vi "ChiSquareCalculation.vi"(2 "Extinction ExtinctionUncertainity Size parameter and Number ofS sizes 2":T2={"Extinction"=[], "Extinction Uncertainty"=[], "Size parameters"=[], "Number ofSizes"=0.0, "GeometricCrossSection"=[], "Wave Length"=0.0, "SMPS Sizes"=[], "Concentration"=[], "Double Charge Correction"=FALSE, "Extincation Factor"=1.0, "Diameter Factor"=1.0, "Diameter Offset"=0.0, "Extinction Factor Flag"=FALSE, "Diameter Factor Flag"=FALSE, "Diameter Offset Flag"=FALSE, "Sizes"=[], "ExtinctionOrAbsorptionOrScattering"=0} {"ExtinctionOrAbsorptionOrScattering" scale=0.0..2.0}, 3 "refractive index, imaginary":sgl=0.1 step=0.01 format="%.3f", 4 "refractive index, real":sgl=1.3 step=0.01 format="%.3f") -> (0 "Normalized Residuals":dbl[](array[numeric]), 1 "Chi Squared":dbl)   [LabVIEW 2011]
uses:
  BaesDataTypeDefinition.ctl
panel:
  out "Extinction Graph":T1(graph)=[{"Ramp Pattern"=[1.7709090992870622, 2.2136363741088276, 2.656363648930593, 3.0990909237523585, 3.5418181985741244, 3.98454547339589, 4.427272748217655], "Extinction"=[2.6163673e-09, 3.3294045e-09, 4.1920147e-09, 4.6714708e-09, 6.2441643e-09, 8.2969445e-09, 9.5108899e-09]}, {"Ramp Pattern"=array[1000 elements], "Extinction"=array[1000 elements]}]
  out "Expected Value For R and I refractive Index":sgl[](array[numeric])
  # "Mie scattering demo program, August 2005, by Martin Fierz (martin@fierz.ch)\n\nThis VI demonstrates the usage of mie2.dll; a dynamic-link-library which you can call in your LabView program.\nThe demo lets you select the refractive index of a sphere, and the size parameter and computes total scattering,\ntotal extinction and angular distribution of the scattered light for p-, s- and unpolarized light.\nMie2.dll uses the Bohren-Huffman Mie code."
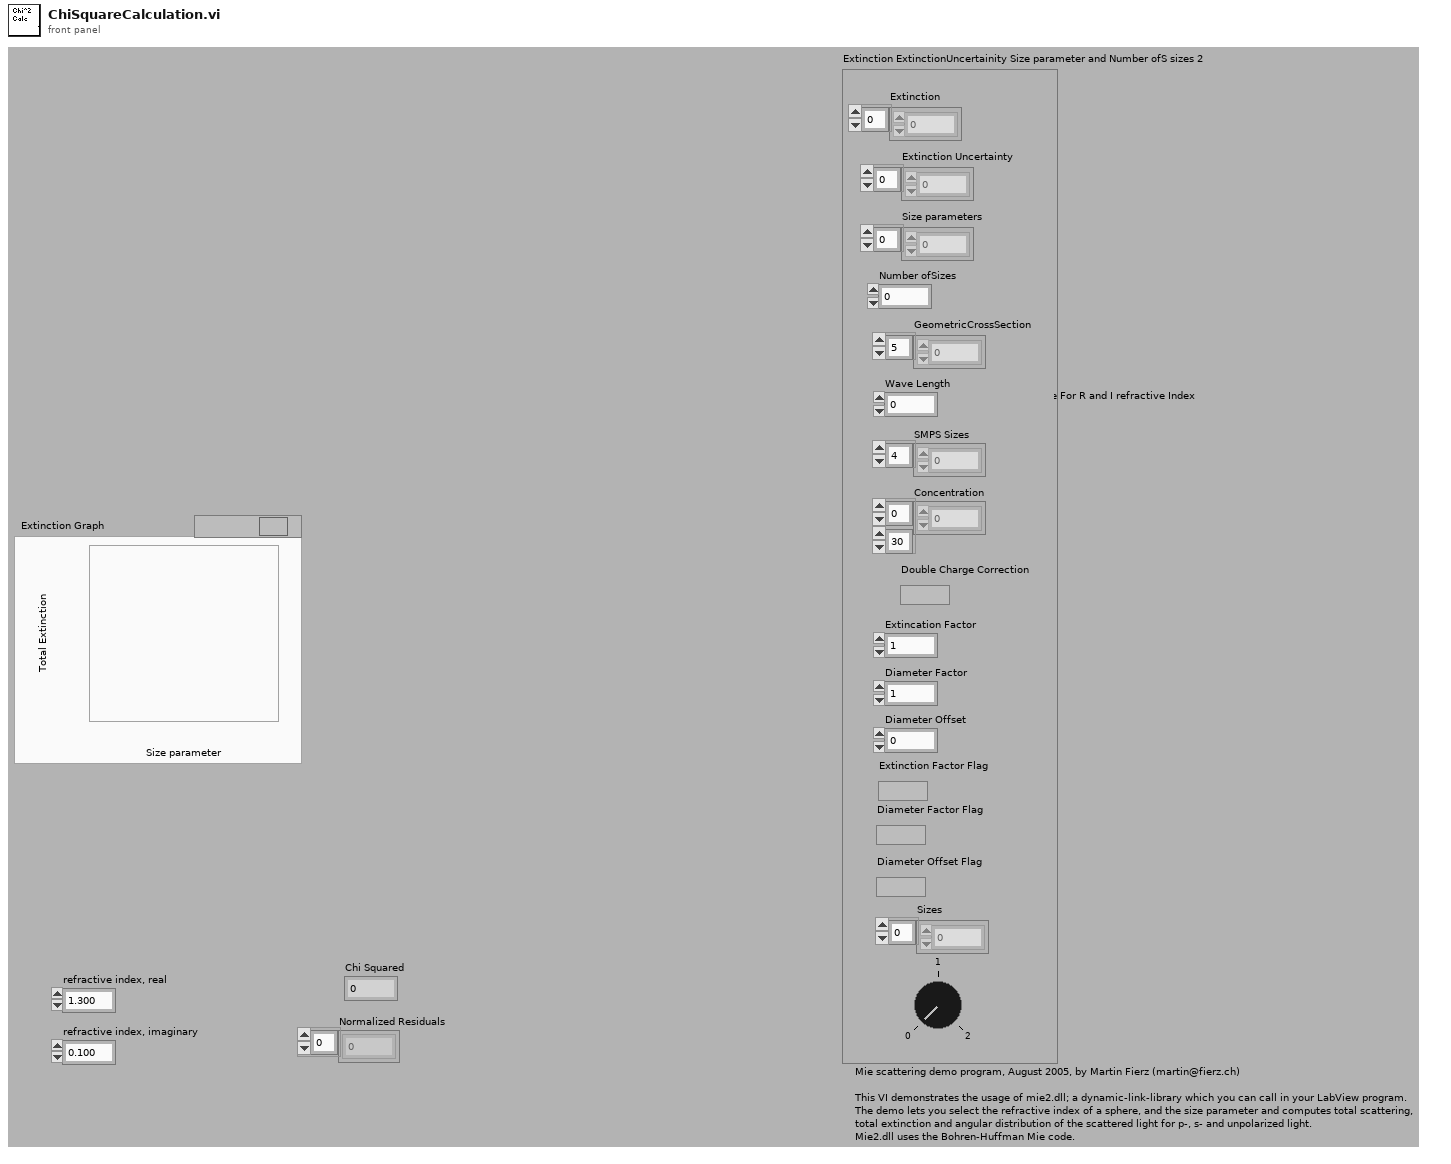
[diagram p1: front panel]
types:
  T1 = cluster{"Ramp Pattern":dbl[], "Extinction":dbl[]}[]
  T2 = typedef "BaesDataTypeDefinition.ctl" = cluster{"Extinction":dbl[], "Extinction Uncertainty":dbl[], "Size parameters":dbl[], "Number ofSizes":dbl, "GeometricCrossSection":dbl[], "Wave Length":dbl, "SMPS Sizes":dbl[], "Concentration":dbl[][], "Double Charge Correction":bool, "Extincation Factor":dbl, "Diameter Factor":dbl, "Diameter Offset":dbl, "Extinction Factor Flag":bool, "Diameter Factor Flag":bool, "Diameter Offset Flag":bool, "Sizes":dbl[], "ExtinctionOrAbsorptionOrScattering":i8}
  T3 = cluster{"Size parameters":dbl[], "Expected Extinction Cross Section":sgl[]}
  T4 = cluster{"Size parameters":dbl[], "Extinction":dbl[]}
  T5 = cluster{"Size parameters":dbl[], "Extinction":dbl[]}[]
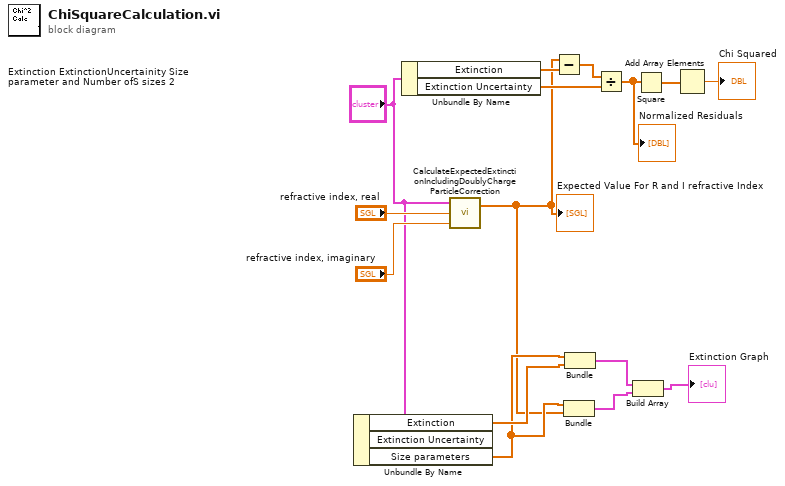
[diagram p0: block diagram]
diagram:
  n1 = Unbundle By Name("Extinction ExtinctionUncertainity Size parameter and Number ofS sizes 2") -> ("Extinction"=w6:dbl[], "Size parameters"=w4:dbl[])  [unwired: 1 out]
  n2 = Unbundle By Name("Extinction ExtinctionUncertainity Size parameter and Number ofS sizes 2") -> ("Extinction"=w11:dbl[], "Extinction Uncertainty"=w10:dbl[])
  n3 = call "CalculateExpectedExtinctionIncludingDoublyChargeParticleCorrection.vi"("refractive index, imaginary"="refractive index, imaginary", "refractive index, real"="refractive index, real", "Extinction ExtinctionUncertainity Size parameter and Number ofS sizes"="Extinction ExtinctionUncertainity Size parameter and Number ofS sizes 2") -> ("Expected Extinction Cross Section"=w3:sgl[])  [unwired: 1 out]
  "Expected Value For R and I refractive Index" <- w3
  n4 = Subtract(x=w3, y=w11) -> (x-y=w15:dbl[])
  n5 = Bundle("Size parameters"=w4, "Expected Extinction Cross Section"=w3) -> (w2:T3)  [unwired: 1 in]
  n6 = Bundle("Size parameters"=w4, "Extinction"=w6) -> (w5:T4)  [unwired: 1 in]
  n7 = Divide(x=w15, y=w10) -> (x/y=w14:dbl[])
  "Normalized Residuals" <- w14
  n8 = Build Array(w5, w2) -> (→"Extinction Graph":T5)
  n9 = Square(x=w14) -> (x^2=w13:dbl[])
  n10 = Add Array Elements(numeric array=w13) -> (sum=→"Chi Squared":dbl)
